vi "SetPin.vi"(0 "MCU in":refnum<class "MCU.lvclass">, 5 "Port":u8, 7 "Pin":u8, 9 "Value":bool, 11 "error in (no error)":errorcluster) -> (4 "MCU out":refnum<class "MCU.lvclass">, 15 "error out":errorcluster)   [LabVIEW 2020, in "MCU.lvclass"]
doc: "Sends a command to write on a pin of the target device."
uses:
  MCU.lvclass
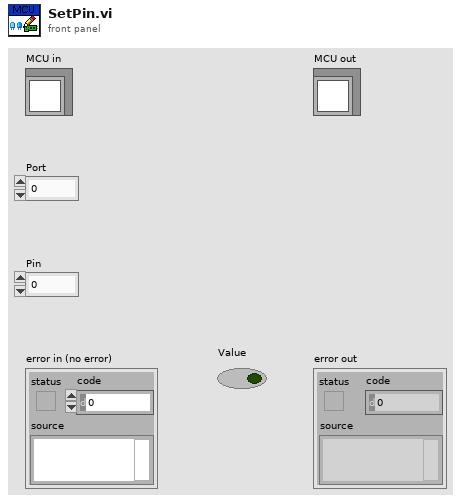
[diagram p1: front panel]
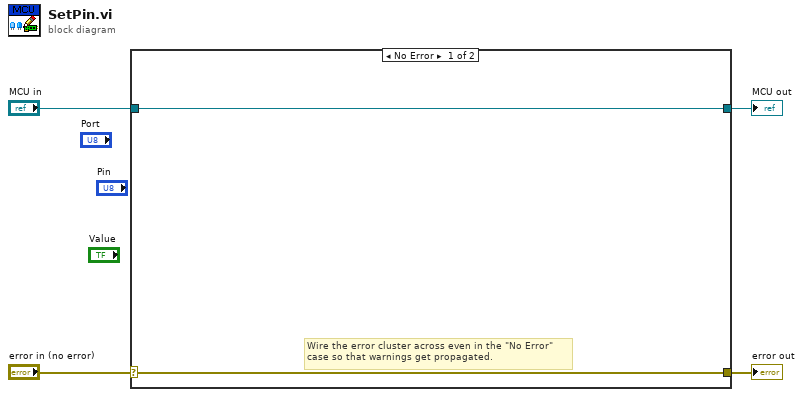
[diagram p0: block diagram]
diagram:
  n1 = case shown="No Error" "error in (no error)" {
    selector: "error in (no error)" -> [w5 w8]
    tunnel: [w5 w8] -> w3
    tunnel: [w6 w7] -> w1
    tunnel: "MCU in" -> [w6 w7]
    frame No Error {
      # "Wire the error cluster across even in the \"No Error\"\ncase so that warnings get propagated."
    }
    frame Error {
    }
  }
  "error out" <- w3
  "MCU out" <- w1
